vi "KE6221 -- Get Square Or Ramp Wave Params.vi"(0 "Resource In":refnum<visa-resource-name>, 1 "Check For SCPI Errors? (T)":bool=TRUE, 11 "error in (no error)":errorcluster) -> (4 "Resource Out (dupl)":refnum<visa-resource-name>, 6 "Wave Type":T1=enum."Square", 8 "Square Or Ramp Wave Params":T2={"Frequency (Hz)"=1000.0, "Amplitude (A)"=0.001, "Offset (A)"=0.0, "Duty Cycle (%)"=50.0, "Ranging Mode"=enum."Best", "Fixed Range"=enum."2mA", "Playback Mode"=enum."Time", "Time (s)"=1.0, "Num Cycles"=1.0, "Phase\nMarker?"=FALSE, "Phase Marker (deg)"=180.0, "Trig Link Line"=enum."1"} {"Duty Cycle (%)" min=0.0 max=100.0 format="%.3p"; "Offset (A)" min=-0.105 max=0.105 format="%.4p"; "Num Cycles" min=0.001 max=99999999900.0 format="%.3p"; "Time (s)" min=1e-07 max=999999.999 format="%.3p"; "Phase Marker (deg)" min=0.0 max=360.0 format="%.3f"; "Amplitude (A)" min=2e-12 max=0.105 format="%.3p"; "Frequency (Hz)" min=0.001 max=100000.0 format="%.3p"}, 15 "error out":errorcluster)   [LabVIEW 2019, in "Keithley 622x.lvlib"]
doc: "Returns the parameters for either a square wave or a ramp wave, in addition to the type of waveform that is currently set for playback (NOTE: this _might not_ be a square wave or ramp wave). Note that this VI can only be used with the 6221, since the 6220 doesn't support this feature."
uses:
  Keithley 622x.lvlib
  Typedefs/KE6221 -- Wave Square Or Ramp Wave Params.ctl
  Low Level/Typedefs/KE6221 -- Wave Frequency.ctl
  Low Level/Typedefs/KE6221 -- Wave Amplitude.ctl
  Source/Typedefs/KE622x -- Current Level.ctl
  Low Level/Typedefs/KE6221 -- Wave Duty Cycle.ctl
  Low Level/Typedefs/KE6221 -- Wave Ranging Mode.ctl
  Source/Typedefs/KE622x -- Current Ranges.ctl
  Low Level/Typedefs/KE6221 -- Wave Playback Mode.ctl
  Low Level/Typedefs/KE6221 -- Wave Playback Time.ctl
  Low Level/Typedefs/KE6221 -- Wave Playback Num Cycles.ctl
  Low Level/Typedefs/KE6221 -- Wave Phase Marker.ctl
  Trigger/Low Level/Typedefs/KE622x -- Trig Link Line.ctl
  Low Level/Typedefs/KE6221 -- Wave Type.ctl
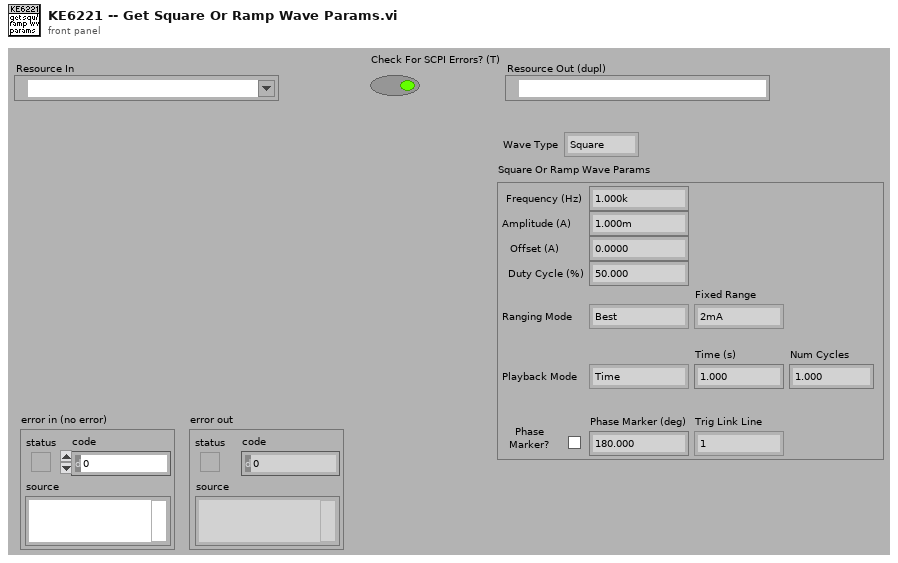
[diagram p1: front panel]
types:
  T1 = typedef "Keithley 622x.lvlib/KE6221 -- Wave Type.ctl" = enum16{"Sinusoid", "Square", "Ramp", "Arbitrary 0", "Arbitrary 1", "Arbitrary 2", "Arbitrary 3", "Arbitrary 4"}
  T2 = typedef "Keithley 622x.lvlib/KE6221 -- Wave Square Or Ramp Wave Params.ctl" = cluster{"Frequency (Hz)":T3, "Amplitude (A)":T4, "Offset (A)":T5, "Duty Cycle (%)":T6, "Ranging Mode":T7, "Fixed Range":T8, "Playback Mode":T9, "Time (s)":T10, "Num Cycles":T11, "Phase\nMarker?":bool, "Phase Marker (deg)":T12, "Trig Link Line":T13}
  T3 = typedef "Keithley 622x.lvlib/KE6221 -- Wave Frequency.ctl" = dbl
  T4 = typedef "Keithley 622x.lvlib/KE6221 -- Wave Amplitude.ctl" = dbl
  T5 = typedef "Keithley 622x.lvlib/KE622x -- Current Level.ctl" = dbl
  T6 = typedef "Keithley 622x.lvlib/KE6221 -- Wave Duty Cycle.ctl" = dbl
  T7 = typedef "Keithley 622x.lvlib/KE6221 -- Wave Ranging Mode.ctl" = enum16{"Best", "Fixed"}
  T8 = typedef "Keithley 622x.lvlib/KE622x -- Current Ranges.ctl" = enum16{"2nA", "20nA", "200nA", "2uA", "20uA", "200uA", "2mA", "20mA", "100mA"}
  T9 = typedef "Keithley 622x.lvlib/KE6221 -- Wave Playback Mode.ctl" = enum16{"Time", "Num Cycles"}
  T10 = typedef "Keithley 622x.lvlib/KE6221 -- Wave Playback Time.ctl" = dbl
  T11 = typedef "Keithley 622x.lvlib/KE6221 -- Wave Playback Num Cycles.ctl" = dbl
  T12 = typedef "Keithley 622x.lvlib/KE6221 -- Wave Phase Marker.ctl" = dbl
  T13 = typedef "Keithley 622x.lvlib/KE622x -- Trig Link Line.ctl" = enum16{"1", "2", "3", "4", "5", "6"}
  T14 = typedef "Keithley 622x.lvlib/KE622x -- Current Range.ctl" = cluster{"Auto Range?":bool, "Man / Selected\nRange":T8}
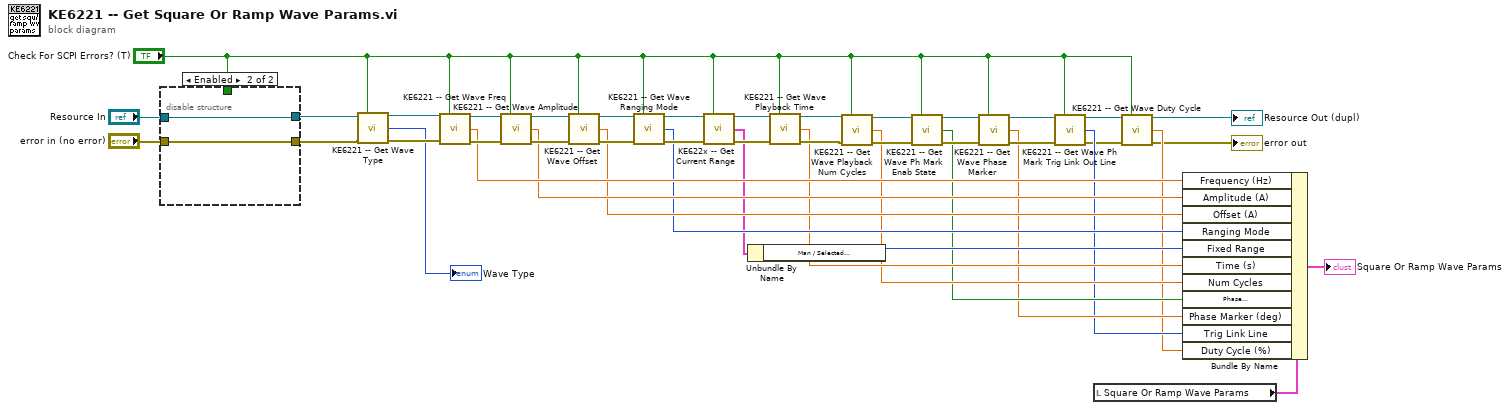
[diagram p0: block diagram]
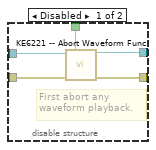
[diagram p2: hidden frame]
diagram:
  n1 = disable-structure shown="Enabled" {
    disable-tunnel: "Resource In" -> [w49 w51]
    disable-tunnel: "error in (no error)" -> [w48 w50]
    disable-tunnel: "Check For SCPI Errors? (T)" -> [w47 _]
    disable-tunnel: [w46 w51] -> w6
    disable-tunnel: [w45 w50] -> w5
    frame Disabled {
      # "First abort any\nwaveform playback."
      n2 = call "KE6221 -- Abort Waveform Func.vi"("Resource In"=w49, "Check For SCPI Errors? (T)"=w47, "error in (no error)"=w48) -> ("Resource Out (dupl)"=w46:refnum<visa-resource-name>, "error out"=w45:errorcluster)  [unwired: 11 in]
    }
    frame Enabled {
    }
  }
  n3 = call "KE6221 -- Get Wave Type.vi"("Resource In"=w6, "Check For SCPI Errors? (T)"="Check For SCPI Errors? (T)", "error in (no error)"=w5) -> ("Resource Out (dupl)"=w4:refnum<visa-resource-name>, "KE6221 Wave Type"=→"Wave Type":T1, "error out"=w3:errorcluster)  [unwired: 10 in]
  n4 = call "KE6221 -- Get Wave Freq.vi"("Resource In"=w4, "Check For SCPI Errors? (T)"="Check For SCPI Errors? (T)", "error in (no error)"=w3) -> ("Resource Out (dupl)"=w44:refnum<visa-resource-name>, "KE6221 Wave Freq (Hz)"=w25:T3, "error out"=w43:errorcluster)  [unwired: 10 in]
  n5 = call "KE6221 -- Get Wave Amplitude.vi"("Resource In"=w44, "Check For SCPI Errors? (T)"="Check For SCPI Errors? (T)", "error in (no error)"=w43) -> ("Resource Out (dupl)"=w40:refnum<visa-resource-name>, "Wave Amplitude"=w24:T4, "error out"=w39:errorcluster)  [unwired: 10 in]
  n6 = call "KE6221 -- Get Wave Offset.vi"("Resource In"=w40, "Check For SCPI Errors? (T)"="Check For SCPI Errors? (T)", "error in (no error)"=w39) -> ("Resource Out (dupl)"=w38:refnum<visa-resource-name>, "Wave Offset (A)"=w23:T5, "error out"=w37:errorcluster)  [unwired: 10 in]
  n7 = call "KE6221 -- Get Wave Ranging Mode.vi"("Resource In"=w38, "Check For SCPI Errors? (T)"="Check For SCPI Errors? (T)", "error in (no error)"=w37) -> ("Resource Out (dupl)"=w42:refnum<visa-resource-name>, "Ranging Mode"=w22:T7, "error out"=w41:errorcluster)  [unwired: 10 in]
  n8 = call "KE622x -- Get Current Range.vi"("Resource In"=w42, "Check For SCPI Errors? (T)"="Check For SCPI Errors? (T)", "error in (no error)"=w41) -> ("Resource Out (dupl)"=w36:refnum<visa-resource-name>, "Current Range"=w21:T14, "error out"=w35:errorcluster)  [unwired: 10 in]
  n9 = Unbundle By Name(w21) -> ("Man / Selected\nRange"=w20:T8)
  n10 = call "KE6221 -- Get Wave Playback Time.vi"("Resource In"=w36, "Check For SCPI Errors? (T)"="Check For SCPI Errors? (T)", "error in (no error)"=w35) -> ("Resource Out (dupl)"=w34:refnum<visa-resource-name>, "Playback Time (s)"=w19:T10, "error out"=w33:errorcluster)  [unwired: 10 in]
  n11 = call "KE6221 -- Get Wave Playback Num Cycles.vi"("Resource In"=w34, "Check For SCPI Errors? (T)"="Check For SCPI Errors? (T)", "error in (no error)"=w33) -> ("Resource Out (dupl)"=w32:refnum<visa-resource-name>, "Num Cycles"=w18:T11, "error out"=w31:errorcluster)  [unwired: 10 in]
  n12 = call "KE6221 -- Get Wave Ph Mark Enab State.vi"("Resource In"=w32, "Check For SCPI Errors? (T)"="Check For SCPI Errors? (T)", "error in (no error)"=w31) -> ("Resource Out (dupl)"=w30:refnum<visa-resource-name>, "Phase Marker Enabled?"=w17:bool, "error out"=w29:errorcluster)  [unwired: 10 in]
  n13 = call "KE6221 -- Get Wave Phase Marker.vi"("Resource In"=w30, "Check For SCPI Errors? (T)"="Check For SCPI Errors? (T)", "error in (no error)"=w29) -> ("Resource Out (dupl)"=w28:refnum<visa-resource-name>, "Phase Marker (deg)"=w16:T12, "error out"=w27:errorcluster)  [unwired: 10 in]
  n14 = call "KE6221 -- Get Wave Ph Mark Trig Link Out Line.vi"("Resource In"=w28, "Check For SCPI Errors? (T)"="Check For SCPI Errors? (T)", "error in (no error)"=w27) -> ("Resource Out (dupl)"=w14:refnum<visa-resource-name>, "Trig Link Out Line"=w15:T13, "error out"=w13:errorcluster)  [unwired: 10 in]
  n15 = local read "Square Or Ramp Wave Params"() -> (w26:T2)
  n16 = call "KE6221 -- Get Wave Duty Cycle.vi"("Resource In"=w14, "Check For SCPI Errors? (T)"="Check For SCPI Errors? (T)", "error in (no error)"=w13) -> ("Resource Out (dupl)"=→"Resource Out (dupl)":refnum<visa-resource-name>, "KE6221 Wave Duty Cycle (%)"=w12:T6, "error out"=→"error out":errorcluster)  [unwired: 10 in]
  n17 = Bundle By Name(cluster=w26, "Frequency (Hz)"=w25, "Amplitude (A)"=w24, "Offset (A)"=w23, "Ranging Mode"=w22, "Fixed Range"=w20, "Time (s)"=w19, "Num Cycles"=w18, "Phase\nMarker?"=w17, "Phase Marker (deg)"=w16, "Trig Link Line"=w15, "Duty Cycle (%)"=w12) -> (→"Square Or Ramp Wave Params":T2)
